vi "Rising Edge 2.vi"(11 "Boolean Array":bool[](array[boolean])) -> (1 "triggered? 3":bool, 2 "triggered? 2":bool, 3 "triggered? 1":bool)   [LabVIEW 2017]
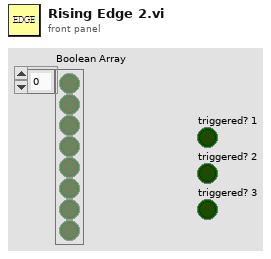
[diagram p1: front panel]
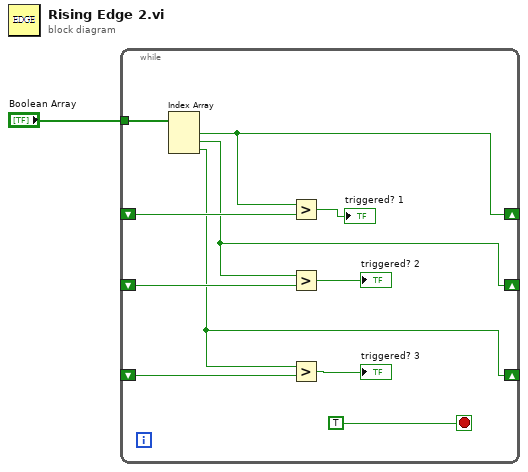
[diagram p0: block diagram]
diagram:
  n1 = while {
    shift-right: [w3] -> _
    shift-left: _ -> [w11]
    tunnel: "Boolean Array" -> [w10]
    shift-right: [w4] -> _
    shift-left: _ -> [w9]
    shift-right: [w2] -> _
    shift-left: _ -> [w8]
    stop <- TRUE stop-if-true
    n2 = Index Array(array=w10) -> (element #1=w4:bool, element #2=w3:bool, element #3=w2:bool)  [unwired: 3 in]
    n3 = Greater?(x=w4, y=w9) -> (0:→"triggered? 1":bool)
    n4 = Greater?(x=w3, y=w11) -> (0:→"triggered? 2":bool)
    n5 = Greater?(x=w2, y=w8) -> (0:→"triggered? 3":bool)
  }
